vi "ROI group-Update groups ctrl.vi"(8 "error in (no error)":errorcluster) -> (0 "error out":errorcluster)   [LabVIEW 2013]
uses:
  ROI Selection Interface/ROI group info cluster.ctl
  Experiment header interface/Typedefs/Save-Load-Save as-Load last enum.ctl
  Typedefs/Group sel cluster.ctl
  Global variables/gl_Functional Imaging-Global variables.vi
panel:
  out "Groups setup":T1[](array[typedef]) {"Group region specifier cluster"."Contours"."Type" items=["No Selection", "Point", "Line", "Rectangle", "Oval", "Polygon", "Freehand Region", "Annulus", "Unused2", "Unused3", "Broken Line", "Freehand Line", "Rotated Rectangle"]}
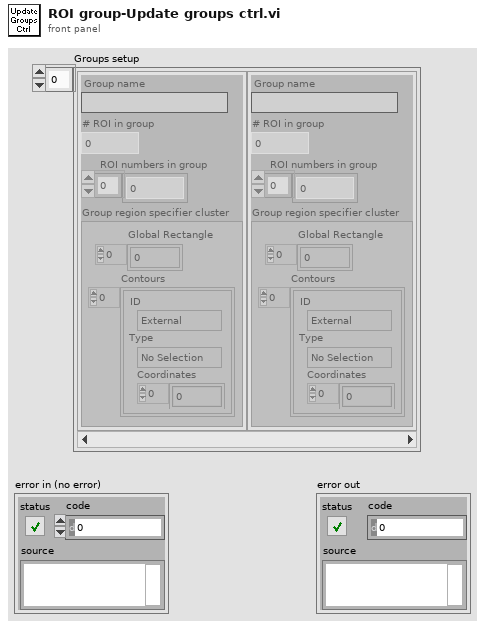
[diagram p1: front panel]
types:
  T1 = typedef "ROI group info cluster.ctl" = cluster{"Group name":string, "# ROI in group":i32, "ROI numbers in group":i32[], "Group region specifier cluster":T2}
  T2 = typedef "ROI Descriptor" = cluster{"Global Rectangle":i32[], "Contours":cluster{"ID":enum32{"External", "Internal"}, "Type":u32, "Coordinates":i32[]}[]}
  T3 = typedef "Save-Load-Save as-Load last enum.ctl" = enum16{"Save file", "Save file as", "Load file", "Load last file"}
  T4 = typedef "Group sel cluster.ctl" = cluster{"Group number":string, "Group Name":string, "Visibility":bool, "Highlight":bool}
  T5 = typedef "Functional Imging UI Refs.ctl" = cluster{"Menu ref":refnum<k9>, "Image control":refnum<vi>, "VI ref":refnum<vi>, "XGrapher":refnum<vi>, "Smoothing":refnum<vi>, "POI Averaging":refnum<vi>, "Normalize":refnum<vi>, "POI data points in each trial":refnum<vi>, "Channel":refnum<vi>, "Experiment data folder path":refnum<vi>, "[ROI vis]":refnum<vi>, "[Groups] visbl":T6, "Group Name":refnum<vi>, "POI index":refnum<vi>, "Trial No.":refnum<vi>, "Intensity Zoom":refnum<vi>, "Trial Cursor Enabled":refnum<vi>, "Number of Trials (ind 1)":refnum<vi>, "Number of Trials (ind 2)":refnum<vi>, "MiniScans Available":refnum<vi>, "POI Available":refnum<vi>, "Defer graph updates":refnum<vi>, "Waveform selector":refnum<vi>, "#of selected POI":refnum<vi>, "#of selected MiniScans":refnum<vi>, "#of selected groups":refnum<vi>, "Max Z-Projection":refnum<vi>, "Z-Plane Selector":refnum<vi>, "Index of miniscan point to visualise":refnum<vi>, "ROI vis. mode":refnum<vi>, "Total # of points":refnum<vi>, "Index of group clicked on":refnum<vi>, "Pane 1":refnum<vi>, "Pane 2":refnum<vi>, "Pane 3":refnum<vi>, "Pane 4":refnum<vi>, "Pane 5":refnum<vi>, "Pane 6":refnum<vi>, "Deselect all ROI":refnum<vi>, "Deselect all groups":refnum<vi>}
  T6 = typedef "Groups array referecne.ctl" = refnum<vi>
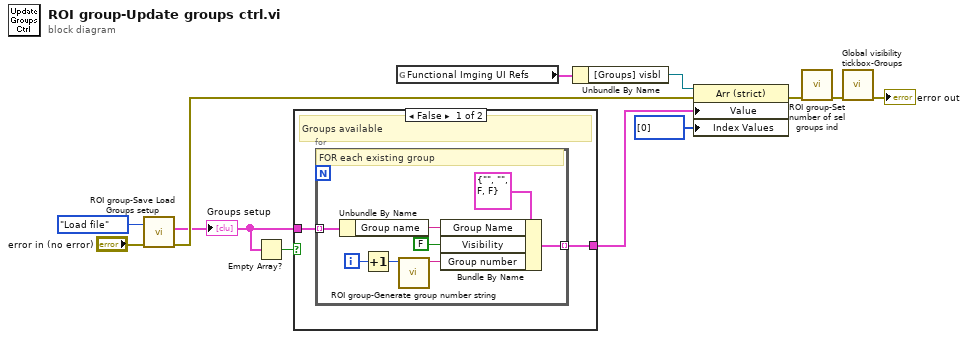
[diagram p0: block diagram]
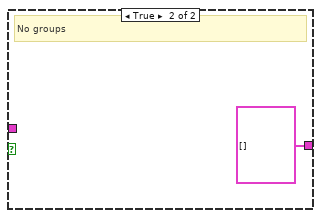
[diagram p2: hidden frame]
diagram:
  n1 = call "ROI group-Save Load Groups setup.vi"("error in (no error)"="error in (no error)", "Function"=Save-Load-Save_as-Load_last_enum."Load file") -> ("error out"=w5:errorcluster, "Loaded groups setup"=w2:T1[])  [unwired: 8 in]
  "Groups setup" <- w2
  n2 = Empty Array?(array=w2) -> (empty?=w1:bool)
  n3 = case shown="False" w1 {
    tunnel: [w14 T4[] []] -> w10
    tunnel: w2 -> [w13 _]
    frame False {
      # "Groups available"
      n4 = for {
        tunnel: w13 -> [w22] mode=indexing
        tunnel: [w20] -> w14 mode=indexing
        i -> [w18]
        # "FOR each existing group"
        n5 = Unbundle By Name(w22) -> ("Group name"=w21:string)
        n6 = Increment(x=w18) -> (x+1=w15:i32)
        n7 = call "ROI group-Generate group number string.vi"("Group number"=w15) -> ("Group number string"=w16:string)  [unwired: 10 in]
        n8 = Bundle By Name(cluster=T4 {"Group number"="", "Group Name"="", "Visibility"=FALSE, "Highlight"=FALSE} ("POI sel & vis"), "Group Name"=w21, "Visibility"=FALSE, "Group number"=w16) -> (w20:T4)
      }
    }
    frame True {
      # "No groups"
    }
  }
  n9 = global read "gl_Functional Imaging-Global variables.vi" "Functional Imging UI Refs"() -> (w8:T5)
  n10 = Unbundle By Name(w8) -> ("[Groups] visbl"=w11:T6)
  n11 = property on="Property Node" class="Arr (strict)"(reference=w11, error in=w5, "Value"=w10, "Index Values"=u32[] [0]) -> (error out=w9:errorcluster)  [unwired: 1 out]
  n12 = call "ROI group-Set number of sel groups ind.vi"("error in (no error)"=w9) -> ("error out"=w4:errorcluster)  [unwired: 10 in]
  n13 = call "Global visibility tickbox-Groups.vi"("error in (no error)"=w4) -> ("error out"=→"error out":errorcluster)  [unwired: 10 in]
